vi "1dArrayTo2dArray.vi"(11 "1D Array":dbl[](array[numeric])) -> (3 "2D Array":dbl[][](array[numeric]))   [LabVIEW 2016]
doc: "Reshape the 1D array to 2D array."
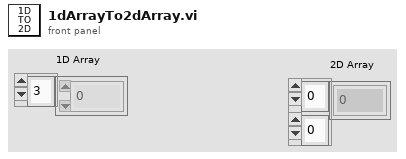
[diagram p1: front panel]
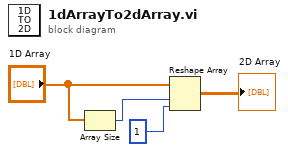
[diagram p0: block diagram]
diagram:
  n1 = Array Size(array="1D Array") -> (size(s)=w1:i32)
  n2 = Reshape Array("1D Array", w1, 1 ("dimension size")) -> (→"2D Array":dbl[][])
